vi "_attribute_read_string.vi"(5 "Repeated Capability":string, 7 "Attribute":T1={"Identifier"="", "Descriptive Name"="", "Data Type"=enum."Integer 32", "Command"="", "Access"=enum."Read/Write", "Range Table"="", "Read Callback"="", "Write Callback"="", "Supported Models"="", "Instrument Options"="", "Index"=0, "OPC Wait"=FALSE, "No Status Check"=FALSE, "Cache Only"=FALSE}, 8 "error in":errorcluster caption="error in (no error)", 10 "Query Parameter":string, 11 "VISA resource name":refnum<visa-resource-name>) -> (0 "error out":errorcluster, 2 "String out":string, 3 "VISA resource name out":refnum<visa-resource-name>)   [LabVIEW 2020, in "Rohde&Schwarz RTx Oscilloscopes.lvlib" / "rsidr_core.lvlib"]
uses:
  rsidr_core.lvlib
  type_Attribute.ctl
  type_Attribute_Data_Type.ctl
  type_ReadWriteAccess.ctl
  Rohde&Schwarz RTx Oscilloscopes.lvlib
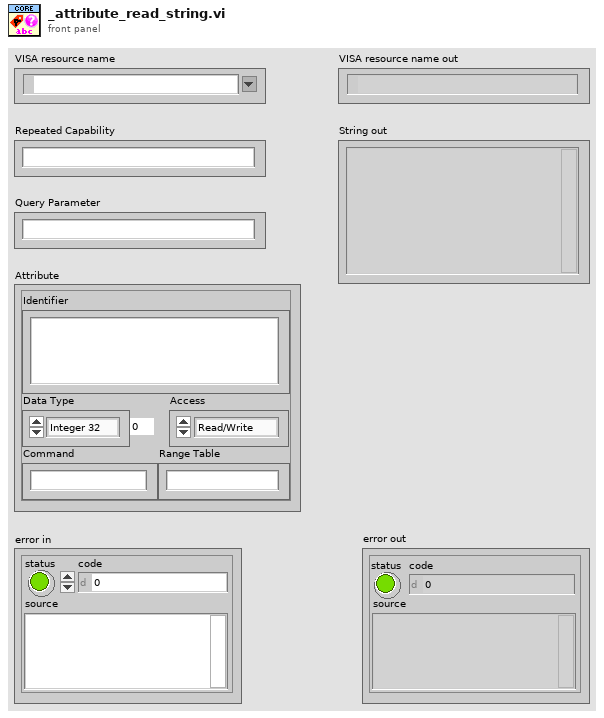
[diagram p1: front panel]
types:
  T1 = typedef "Rohde&Schwarz RTx Oscilloscopes.lvlib/rsidr_core.lvlib/type_Attribute.ctl" = cluster{"Identifier":string, "Descriptive Name":string, "Data Type":T2, "Command":string, "Access":T3, "Range Table":string, "Read Callback":string, "Write Callback":string, "Supported Models":string, "Instrument Options":string, "Index":i32, "OPC Wait":bool, "No Status Check":bool, "Cache Only":bool}
  T2 = typedef "Rohde&Schwarz RTx Oscilloscopes.lvlib/rsidr_core.lvlib/type_Attribute_Data_Type.ctl" = enum16{"Integer 32", "Double", "String", "Boolean", "None", "Integer 64", "RawString"}
  T3 = typedef "Rohde&Schwarz RTx Oscilloscopes.lvlib/rsidr_core.lvlib/type_ReadWriteAccess.ctl" = enum16{"Read Only", "Write Only", "Read/Write"}
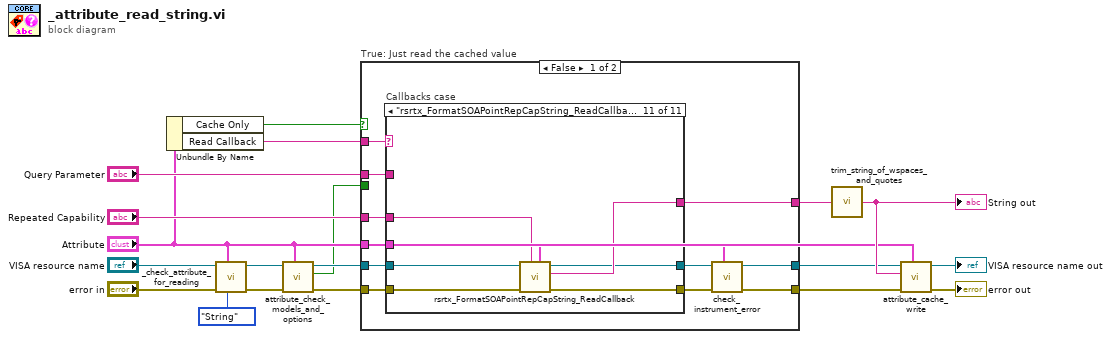
[diagram p0: block diagram]
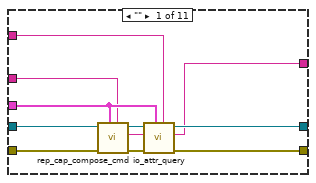
[diagram p2: hidden frame]
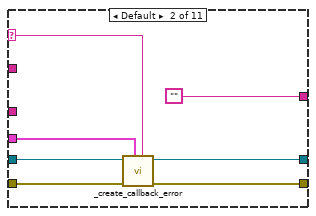
[diagram p3: hidden frame]
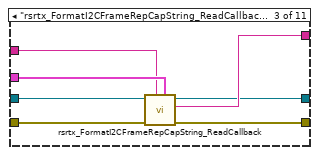
[diagram p4: hidden frame]
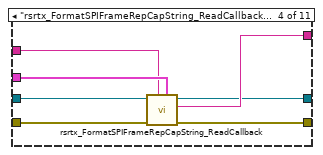
[diagram p5: hidden frame]
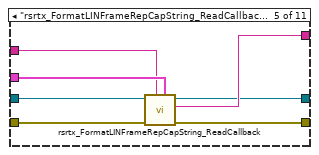
[diagram p6: hidden frame]
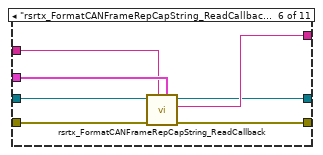
[diagram p7: hidden frame]
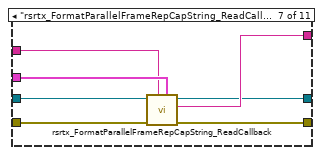
[diagram p8: hidden frame]
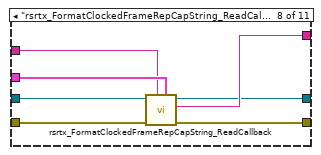
[diagram p9: hidden frame]
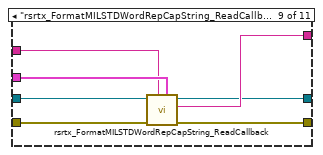
[diagram p10: hidden frame]
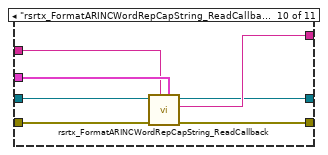
[diagram p11: hidden frame]
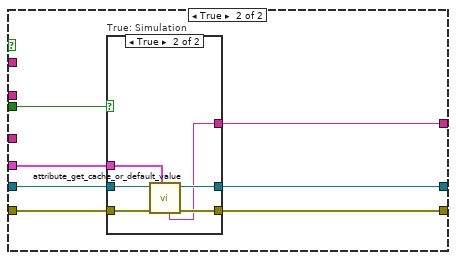
[diagram p12: hidden frame]
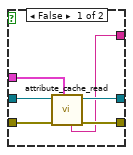
[diagram p13: hidden frame]
diagram:
  n1 = Unbundle By Name("Attribute") -> ("Cache Only"=w1:bool, "Read Callback"=w10:string)
  n2 = call "_check_attribute_for_reading.vi"("Expected Data Type"=type_Attribute_Data_Type."String" ("Data Type"), "Attribute"="Attribute", "error in"="error in", "VISA resource name"="VISA resource name") -> ("error out"=w7:errorcluster, "VISA resource name out"=w6:refnum<visa-resource-name>)  [unwired: 6 in]
  n3 = call "attribute_check_models_and_options.vi"("Attribute"="Attribute", "error in"=w7, "VISA resource name"=w6) -> ("error out"=w5:errorcluster, "Simulation Mode"=w2:bool, "VISA resource name out"=w4:refnum<visa-resource-name>)  [unwired: 6 in]
  n4 = case "True: Just read the cached value" shown="False" w1 {
    tunnel: "Repeated Capability" -> [w30 _]
    tunnel: [w22 w114] -> w9
    tunnel: [w21 w115] -> w8
    tunnel: [w29 w113] -> w13
    tunnel: w10 -> [w28 _]
    tunnel: w4 -> [w27 w118]
    tunnel: w5 -> [w26 w116]
    tunnel: "Attribute" -> [w20 w117]
    tunnel: "Query Parameter" -> [w25 _]
    tunnel: w2 -> [_ w112]
    frame False {
      n5 = case "Callbacks case" shown="\"rsrtx_FormatSOAPointRepCapString_ReadCallback.vi\"" w28 {
        selector: w28 -> [_ w44 _ _ _ _ _ _ _ _ _]
        tunnel: w27 -> [w41 w47 w54 w61 w68 w75 w82 w89 w96 w103 w110]
        tunnel: w26 -> [w40 w48 w55 w62 w69 w76 w83 w90 w97 w104 w111]
        tunnel: w30 -> [w33 _ w52 w59 w66 w73 w80 w87 w94 w101 w108]
        tunnel: [w39 w45 w49 w56 w63 w70 w77 w84 w91 w98 w105] -> w23
        tunnel: [w38 w46 w50 w57 w64 w71 w78 w85 w92 w99 w106] -> w24
        tunnel: [w32 "" ("Empty String Constant") w51 w58 w65 w72 w79 w86 w93 w100 w107] -> w29
        tunnel: w20 -> [w34 w43 w53 w60 w67 w74 w81 w88 w95 w102 w109]
        tunnel: w25 -> [w31 _ _ _ _ _ _ _ _ _ _]
        frame "" {
          n6 = call "rep_cap_compose_cmd.vi"("Repeated Capability"=w33, "Attribute"=w34, "error in"=w40, "VISA resource name"=w41) -> ("error out"=w37:errorcluster, "Command out"=w36:string, "VISA resource name out"=w35:refnum<visa-resource-name>)  [unwired: 5 in]
          n7 = call "io_attr_query.vi"("Query Parameter (None)"=w31, "Attribute"=w34, "error in"=w37, "write buffer"=w36, "VISA resource name"=w35) -> ("error out"=w38:errorcluster, "read buffer"=w32:string, "VISA resource name out"=w39:refnum<visa-resource-name>)  [unwired: 4 in]
        }
        frame Default {
          n8 = call "_create_callback_error.vi"("Callback Name"=w44, "Attribute"=w43, "error in"=w48, "VISA resource name"=w47) -> ("error out"=w46:errorcluster, "VISA resource name out"=w45:refnum<visa-resource-name>)  [unwired: 6 in]
        }
        frame "rsrtx_FormatI2CFrameRepCapString_ReadCallback.vi" {
          n9 = call "rsrtx_FormatI2CFrameRepCapString_ReadCallback.vi"("Attribute"=w53, "Repeated Capability"=w52, "error in"=w55, "VISA resource name"=w54) -> ("error out"=w50:errorcluster, "Attribute Value String"=w51:string, "VISA resource name out"=w49:refnum<visa-resource-name>)  [unwired: 5 in]
        }
        frame "rsrtx_FormatSPIFrameRepCapString_ReadCallback.vi" {
          n10 = call "rsrtx_FormatSPIFrameRepCapString_ReadCallback.vi"("Attribute"=w60, "Repeated Capability"=w59, "error in"=w62, "VISA resource name"=w61) -> ("error out"=w57:errorcluster, "Attribute Value String"=w58:string, "VISA resource name out"=w56:refnum<visa-resource-name>)  [unwired: 5 in]
        }
        frame "rsrtx_FormatLINFrameRepCapString_ReadCallback.vi" {
          n11 = call "rsrtx_FormatLINFrameRepCapString_ReadCallback.vi"("Attribute"=w67, "Repeated Capability"=w66, "error in"=w69, "VISA resource name"=w68) -> ("error out"=w64:errorcluster, "Attribute Value String"=w65:string, "VISA resource name out"=w63:refnum<visa-resource-name>)  [unwired: 5 in]
        }
        frame "rsrtx_FormatCANFrameRepCapString_ReadCallback.vi" {
          n12 = call "rsrtx_FormatCANFrameRepCapString_ReadCallback.vi"("Attribute"=w74, "Repeated Capability"=w73, "error in"=w76, "VISA resource name"=w75) -> ("error out"=w71:errorcluster, "Attribute Value String"=w72:string, "VISA resource name out"=w70:refnum<visa-resource-name>)  [unwired: 5 in]
        }
        frame "rsrtx_FormatParallelFrameRepCapString_ReadCallback.vi" {
          n13 = call "rsrtx_FormatParallelFrameRepCapString_ReadCallback.vi"("Attribute"=w81, "Repeated Capability"=w80, "error in"=w83, "VISA resource name"=w82) -> ("error out"=w78:errorcluster, "Attribute Value String"=w79:string, "VISA resource name out"=w77:refnum<visa-resource-name>)  [unwired: 5 in]
        }
        frame "rsrtx_FormatClockedFrameRepCapString_ReadCallback.vi" {
          n14 = call "rsrtx_FormatClockedFrameRepCapString_ReadCallback.vi"("Attribute"=w88, "Repeated Capability"=w87, "error in"=w90, "VISA resource name"=w89) -> ("error out"=w85:errorcluster, "Attribute Value String"=w86:string, "VISA resource name out"=w84:refnum<visa-resource-name>)  [unwired: 5 in]
        }
        frame "rsrtx_FormatMILSTDWordRepCapString_ReadCallback.vi" {
          n15 = call "rsrtx_FormatMILSTDWordRepCapString_ReadCallback.vi"("Attribute"=w95, "Repeated Capability"=w94, "error in"=w97, "VISA resource name"=w96) -> ("error out"=w92:errorcluster, "Attribute Value String"=w93:string, "VISA resource name out"=w91:refnum<visa-resource-name>)  [unwired: 5 in]
        }
        frame "rsrtx_FormatARINCWordRepCapString_ReadCallback.vi" {
          n16 = call "rsrtx_FormatARINCWordRepCapString_ReadCallback.vi"("Attribute"=w102, "Repeated Capability"=w101, "error in"=w104, "VISA resource name"=w103) -> ("error out"=w99:errorcluster, "Attribute Value String"=w100:string, "VISA resource name out"=w98:refnum<visa-resource-name>)  [unwired: 5 in]
        }
        frame "rsrtx_FormatSOAPointRepCapString_ReadCallback.vi" {
          n17 = call "rsrtx_FormatSOAPointRepCapString_ReadCallback.vi"("Attribute"=w109, "Repeated Capability"=w108, "error in"=w111, "VISA resource name"=w110) -> ("error out"=w106:errorcluster, "Attribute Value String"=w107:string, "VISA resource name out"=w105:refnum<visa-resource-name>)  [unwired: 5 in]
        }
      }
      n18 = call "check_instrument_error.vi"("Attribute"=w20, "error in"=w24, "VISA resource name"=w23) -> ("error out"=w22:errorcluster, "VISA resource name out"=w21:refnum<visa-resource-name>)  [unwired: 7 in]
    }
    frame True {
      n19 = case "True: Simulation" shown="True" w112 {
        tunnel: w116 -> [w124 w130]
        tunnel: w118 -> [w123 w129]
        tunnel: w117 -> [w122 w126]
        tunnel: [w121 w128] -> w114
        tunnel: [w120 w127] -> w115
        tunnel: [w119 w125] -> w113
        frame False {
          n20 = call "attribute_cache_read.vi"("Attribute"=w122, "error in"=w124, "VISA resource name"=w123) -> ("error out"=w121:errorcluster, "VISA resource name out"=w120:refnum<visa-resource-name>, "String out"=w119:string)  [unwired: 1 in, 5 out]
        }
        frame True {
          n21 = call "attribute_get_cache_or_default_value.vi"("Attribute"=w126, "error in"=w130, "VISA resource name"=w129) -> ("error out"=w128:errorcluster, "VISA resource name out"=w127:refnum<visa-resource-name>, "String out"=w125:string)  [unwired: 1 in, 5 out]
        }
      }
    }
  }
  n22 = call "trim_string_of_wspaces_and_quotes.vi"("String in"=w13) -> ("String out"=w12:string)  [unwired: 4 in]
  "String out" <- w12
  n23 = call "attribute_cache_write.vi"("Attribute"="Attribute", "error in"=w9, "Value in"=w12, "VISA resource name"=w8) -> ("error out"=→"error out":errorcluster, "VISA resource name out"=→"VISA resource name out":refnum<visa-resource-name>)  [unwired: 6 in]
